vi "init runtime test.vi"() -> ()   [LabVIEW 2013, in "Modbus Slave tests.lvlib"]
doc: "Platypus Framework 1.0.1.65\nNI Systems Engineering - National Instruments"
uses:
  Modbus Slave tests.lvlib
  <vilib>/NI/Tag Bus/dictionary/data dictionary.lvclass
  execution/Modbus Slave runtime.lvclass
  module channel/Modbus Module Channel.lvclass
panel:
  out "tags found":bool
  out "no error":errorcluster
  out "expected execution settings":bool
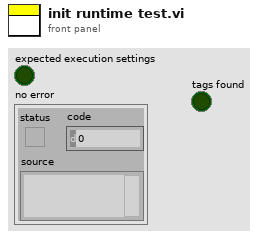
[diagram p1: front panel]
types:
  T1 = typedef "TBM channel.lvclass/data tables.ctl" = cluster{"input data":T2, "processing parameter":T2, "processing result":T2, "output data":T2}
  T2 = typedef "tag bus.lvlib/dictionary table pair.ctl" = cluster{"data dictionary":refnum<class "data dictionary.lvclass">, "data table":T3}
  T3 = typedef "tag bus.lvlib/data table.lvlib/data table.ctl" = cluster{"Double":dbl[], "Single":sgl[], "I64":i64[], "I32":i32[], "I16":i16[], "I8":i8[], "U64":u64[], "U32":u32[], "U16":u16[], "U8":u8[], "Boolean":bool[], "String":string[], "Array of Double":cluster{"DBL Array":dbl[]}[], "Array of Single":cluster{"SGL Array":sgl[]}[], "Array of I64":cluster{"I64 Array":i64[]}[], "Array of I32":cluster{"I32 Array":i32[]}[], "Array of I16":cluster{"I16 Array":i16[]}[], "Array of I8":cluster{"I8 Array":i8[]}[], "Array of U64":cluster{"U64 Array":u64[]}[], "Array of U32":cluster{"U32 Array":u32[]}[], "Array of U16":cluster{"U16 Array":u16[]}[], "Array of U8":cluster{"U8 Array":u8[]}[], "Array of Boolean":cluster{"Boolean Array":bool[]}[], "Array of String":cluster{"String Array":string[]}[]}
  T4 = typedef "TBM module execution interface.lvclass/execution settings.ctl" = cluster{"reads inputs":bool, "processes data":bool, "writes outputs":bool}
  T5 = typedef "tag bus.lvlib/tag descriptor.lvclass/Data Type.ctl" = enum16{"Double", "Single", "I64", "I32", "I16", "I8", "U64", "U32", "U16", "U8", "Boolean", "String", "Array of Double", "Array of Single", "Array of I64", "Array of I32", "Array of I16", "Array of I8", "Array of U64", "Array of U32", "Array of U16", "Array of U8", "Array of Boolean", "Array of String"}
  T6 = typedef "TBM channel.lvclass/channel classification.ctl" = enum16{"input data", "output data", "processing parameter", "processing result"}
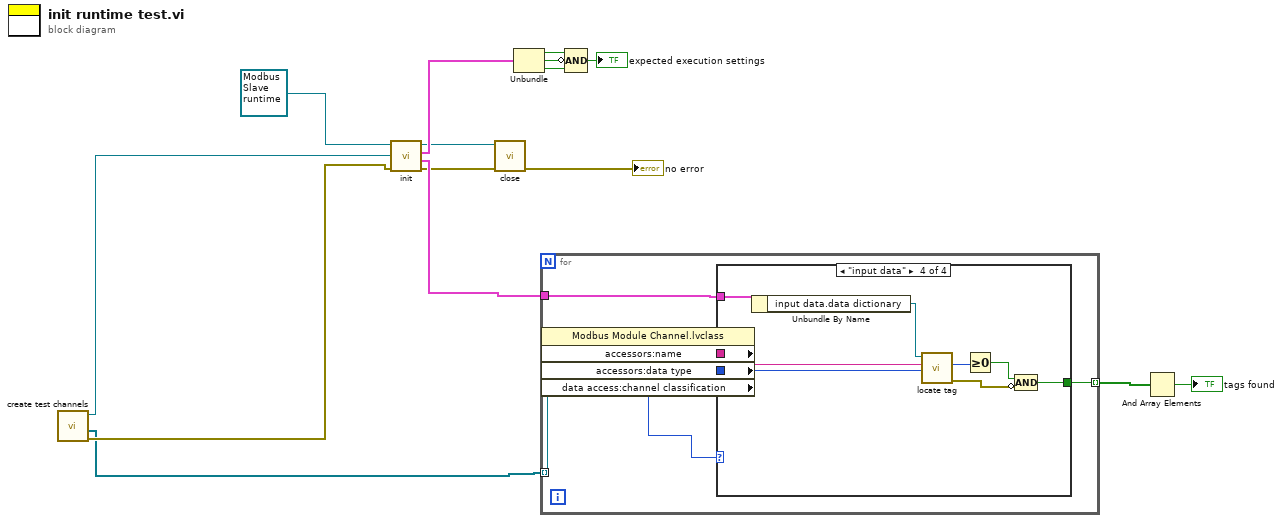
[diagram p0: block diagram]
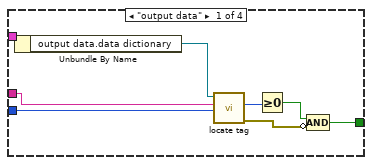
[diagram p2: hidden frame]
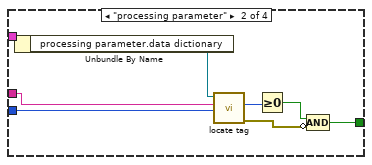
[diagram p3: hidden frame]
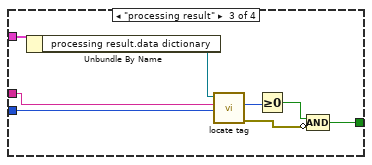
[diagram p4: hidden frame]
diagram:
  n1 = call "create test channels.vi"() -> ("error out"=w2:errorcluster, "Array"=w1:refnum<class "Modbus Module Channel.lvclass">[], "Modbus Slave configuration out"=w3:refnum<class "Modbus Slave configuration.lvclass">)  [unwired: 7 in, 2 out]
  n2 = call-dynamic "init.vi"("error in"=w2, "TBM module configuration in"=w3, "Modbus Slave runtime in"=refnum<class "Modbus Slave runtime.lvclass"> refnum ("tag bus configurable plugin module")) -> ("error out"=w7:errorcluster, "data allocations"=w15:T1, "execution settings"=w14:T4, "Modbus Slave runtime out"=w6:refnum<class "Modbus Slave runtime.lvclass">)  [unwired: 5 in]
  n3 = call-dynamic "close.vi"("error in"=w7, "Modbus Slave runtime in"=w6) -> ("error out"=→"no error":errorcluster)  [unwired: 9 in]
  n4 = Unbundle(w14) -> ("reads inputs"=w13:bool, "processes data"=w11:bool, "writes outputs"=w12:bool)
  n5 = for {
    tunnel: w15 -> [w19]
    tunnel: w1 -> [w21] mode=indexing
    tunnel: [w16] -> w9 mode=indexing
    n6 = property class="Modbus Module Channel.lvclass"(reference=w21) -> ("accessors:name"=w17:string, "accessors:data type"=w18:T5, "data access:channel classification"=w20:T6)  [unwired: 1 in, 2 out]
    n7 = case shown="\"input data\"" w20 {
      tunnel: w19 -> [w29 w37 w45 w53]
      tunnel: w18 -> [w27 w35 w43 w51]
      tunnel: w17 -> [w26 w34 w42 w50]
      tunnel: [w22 w30 w38 w46] -> w16
      frame "output data" {
        n8 = Unbundle By Name(w29) -> ("output data.data dictionary"=w28:refnum<class "data dictionary.lvclass">)
        n9 = call <vilib>:"locate tag.vi"("data type"=w27, "name"=w26, "data dictionary in"=w28) -> ("error out"=w23:errorcluster, "index"=w25:i32)  [unwired: 6 in, 1 out]
        n10 = Greater Or Equal To 0?(x=w25) -> (x >= 0?=w24:bool)
        n11 = Compound Arithmetic op=AND(w24, invert w23) -> (w22:bool)
      }
      frame "processing parameter" {
        n12 = Unbundle By Name(w37) -> ("processing parameter.data dictionary"=w36:refnum<class "data dictionary.lvclass">)
        n13 = call <vilib>:"locate tag.vi"("data type"=w35, "name"=w34, "data dictionary in"=w36) -> ("error out"=w31:errorcluster, "index"=w33:i32)  [unwired: 6 in, 1 out]
        n14 = Greater Or Equal To 0?(x=w33) -> (x >= 0?=w32:bool)
        n15 = Compound Arithmetic op=AND(w32, invert w31) -> (w30:bool)
      }
      frame "processing result" {
        n16 = Unbundle By Name(w45) -> ("processing result.data dictionary"=w44:refnum<class "data dictionary.lvclass">)
        n17 = call <vilib>:"locate tag.vi"("data type"=w43, "name"=w42, "data dictionary in"=w44) -> ("error out"=w39:errorcluster, "index"=w41:i32)  [unwired: 6 in, 1 out]
        n18 = Greater Or Equal To 0?(x=w41) -> (x >= 0?=w40:bool)
        n19 = Compound Arithmetic op=AND(w40, invert w39) -> (w38:bool)
      }
      frame "input data" {
        n20 = Unbundle By Name(w53) -> ("input data.data dictionary"=w52:refnum<class "data dictionary.lvclass">)
        n21 = call <vilib>:"locate tag.vi"("data type"=w51, "name"=w50, "data dictionary in"=w52) -> ("error out"=w47:errorcluster, "index"=w49:i32)  [unwired: 6 in, 1 out]
        n22 = Greater Or Equal To 0?(x=w49) -> (x >= 0?=w48:bool)
        n23 = Compound Arithmetic op=AND(w48, invert w47) -> (w46:bool)
      }
    }
  }
  n24 = Compound Arithmetic op=AND(w13, invert w11, w12) -> (→"expected execution settings":bool)
  n25 = And Array Elements(Boolean array=w9) -> (logical AND=→"tags found":bool)
